vi "LUT_ScoreNumbers.vi"() -> (0 "Init Data Out":fxp<+,4,4>[](array[numeric]))   [LabVIEW 2018]
panel:
  out "1/4":i32
  out "number of columns":i32
  out "number of rows":i32
  out "Original":picture
  out "Quotient":i32
  out "Remainder (Must be 0)":i32
  out "TotalPixels":i32
  out "Init Data Out size":i32
  # "For Initialization VI requirements and help, please read directions located on Block Diagram."
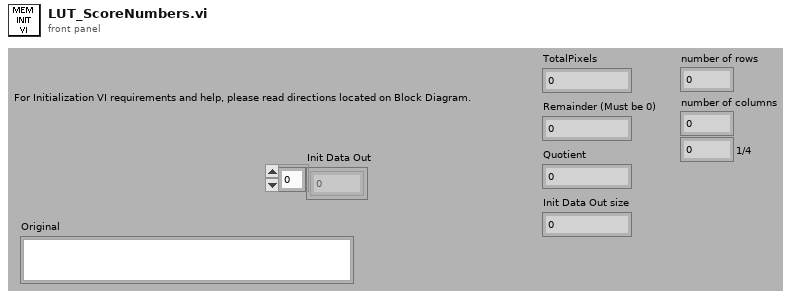
[diagram p1: front panel]
types:
  T1 = typedef "imagedata.ctl" = cluster{"image type":i32, "image depth":i32, "image":u8[], "mask":u8[], "colors":u32[], "Rectangle":cluster{"left":i16, "top":i16, "right":i16, "bottom":i16}}
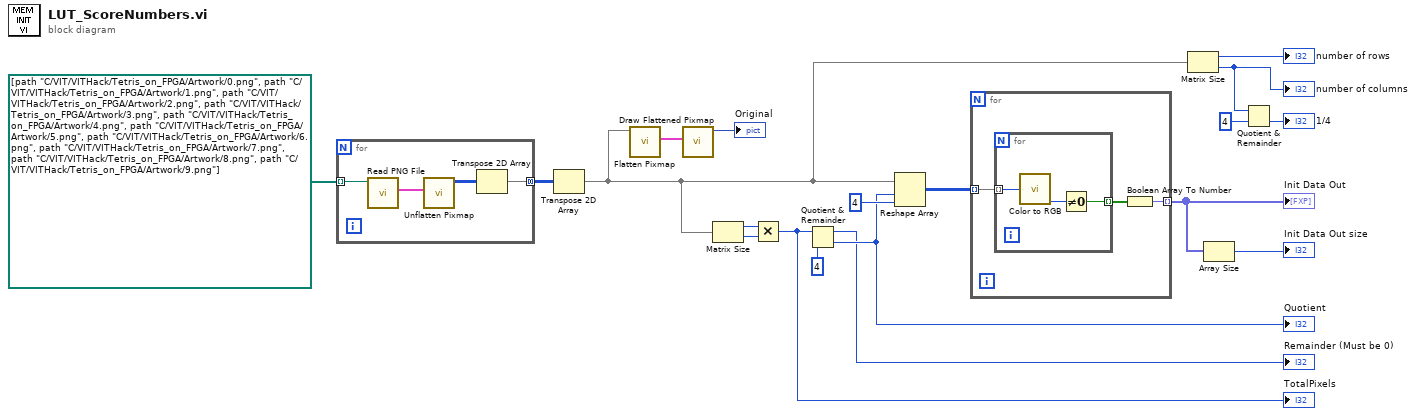
[diagram p0: block diagram]
diagram:
  n1 = for {
    tunnel: [w20] -> w2 mode=concatenating
    tunnel: path[] [path "C:/VIT/VITHack/Tetris_on_FPGA/Artwork/0.png", path "C:/VIT/VITHack/Tetris_on_FPGA/Artwork/1.png", path "C:/VIT/VITHack/Tetris_on_FPGA/Artwork/2.png", path "C:/VIT/VITHack/Tetris_on_FPGA/Artwork/3.png", path "C:/VIT/VITHack/Tetris_on_FPGA/Artwork/4.png", path "C:/VIT/VITHack/Tetris_on_FPGA/Artwork/5.png", path "C:/VIT/VITHack/Tetris_on_FPGA/Artwork/6.png", path "C:/VIT/VITHack/Tetris_on_FPGA/Artwork/7.png", path "C:/VIT/VITHack/Tetris_on_FPGA/Artwork/8.png", path "C:/VIT/VITHack/Tetris_on_FPGA/Artwork/9.png"] -> [w22] mode=indexing
    n2 = call <vilib>:"Read PNG File.vi"("path to PNG file"=w22) -> ("image data"=w23:T1)  [unwired: 8 in, 2 out]
    n3 = call <vilib>:"Unflatten Pixmap.vi"("image data"=w23) -> ("24-bit pixmap"=w21:u32[][])  [unwired: 4 in, 6 out]
    n4 = Transpose 2D Array(2D array=w21) -> (transposed array=w20:u32[][])
  }
  n5 = Transpose 2D Array(2D array=w2) -> (transposed array=w1:u32[][])
  n6 = call <vilib>:"Flatten Pixmap.vi"("24-bit pixmap"=w1) -> ("image data"=w5:T1)  [unwired: 10 in]
  n7 = call <vilib>:"Draw Flattened Pixmap.vi"("image data"=w5) -> ("new picture"=→"Original":picture)  [unwired: 8 in]
  n8 = Matrix Size(0:w1) -> (1:w13:i32, 2:w12:i32)
  n9 = Multiply(x=w13, y=w12) -> (x*y=w18:i32)
  "TotalPixels" <- w18
  n10 = Quotient & Remainder(x=w18, y=4) -> (x-y*floor(x/y)=→"Remainder (Must be 0)":i32, floor(x/y)=w16:i32)
  "Quotient" <- w16
  n11 = Reshape Array(w1, w16, 4 ("dimension size")) -> (w10:u32[][])
  n12 = for {
    tunnel: w10 -> [w26] mode=indexing
    tunnel: [w25] -> w11 mode=indexing
    n13 = for {
      tunnel: w26 -> [w29] mode=indexing
      tunnel: [w27] -> w24 mode=indexing
      n14 = call <vilib>:"Color to RGB.vi"("Color"=w29) -> ("B"=w28:u8)  [unwired: 3 out]
      n15 = Not Equal To 0?(x=w28) -> (x != 0?=w27:bool)
    }
    n16 = Boolean Array To Number(Boolean array=w24) -> (number=w25:fxp<+,4,4>)
  }
  "Init Data Out" <- w11
  n17 = Matrix Size(0:w1) -> (1:→"number of rows":i32, 2:w8:i32)
  "number of columns" <- w8
  n18 = Array Size(array=w11) -> (size(s)=→"Init Data Out size":i32)
  n19 = Quotient & Remainder(x=w8, y=4) -> (floor(x/y)=→"1/4":i32)  [unwired: 1 out]
